vi "sedSpectrometer_monitorCommand_enable.vi"(8 "error in (no error)":errorcluster, 11 "command_enable_Ctl":T1) -> (0 "error out":errorcluster, 2 "function return":i32, 3 "command_enable_Ctl out":T1)   [LabVIEW 2016, in "SALLV_sedSpectrometer.lvlib"]
doc: "int sedSpectrometer_shm_monitorCommand_enableLV(sedSpectrometer_command_enableLV *command_enable_Ctl );"
uses:
  SALLV_sedSpectrometer.lvlib
  DataTypes/command_enable.ctl
  SALLV_sedSpectrometer.so
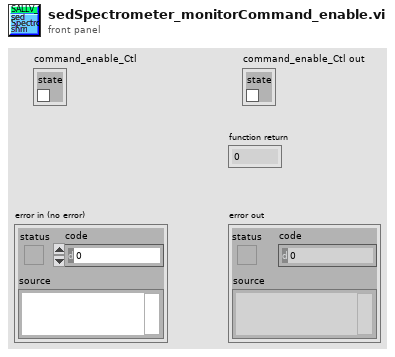
[diagram p1: front panel]
types:
  T1 = typedef "SALLV_sedSpectrometer.lvlib/command_enable.ctl" = cluster{"state":bool}
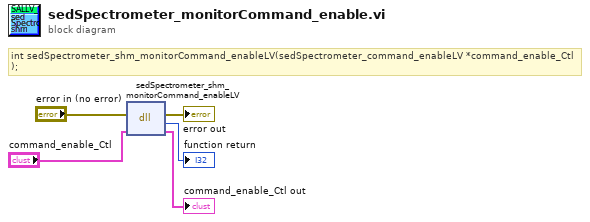
[diagram p0: block diagram]
diagram:
  # "int sedSpectrometer_shm_monitorCommand_enableLV(sedSpectrometer_command_enableLV *command_enable_Ctl );"
  n1 = dll-call lib="home/harini/TCS/SALLV_sedSpectrometer/SALLV_sedSpectrometer.*" fn="sedSpectrometer_shm_monitorCommand_enableLV"(error in="error in (no error)", "command_enable_Ctl"="command_enable_Ctl") -> (error out=→"error out":errorcluster, →"function return":i32, "command_enable_Ctl"=→"command_enable_Ctl out":T1)  [unwired: 2 in, 1 out]
